vi "Test Dynamic Passing Method.vi"(8 "error in (no error)":errorcluster, 11 "Test Test Case in":refnum<class "Test Test Case.lvclass">) -> (0 "error out":errorcluster, 3 "Test Test Case out":refnum<class "Test Test Case.lvclass">)   [LabVIEW 2020, in "Test Test Case.lvclass"]
uses:
  Test Test Case.lvclass
  C:/Git/astemes-lunit/source/Framework/Test Case/LUnit Test Case.lvclass
  source/Framework/Test Case/LUnit Test Case.lvclass/LUnit Test Case.ctl
  source/Framework/Test Case/Private/SubVIs/Add test result.vi
  source/Framework/Test Case/Private/SubVIs/Set Assertion Type.vi
  source/Framework/Result Types/Case Result/Public/Record Assertion Result.vi
  source/Framework/Result Types/Method Result/Public/Aggregate Assertion Results.vi
  source/Framework/Result Types/Method Result/Private/Merge Status.vi
  source/Framework/Result Types/Method Result/Private/Concatenate result strings.vi
  source/Framework/Test Case/LUnit Test Case.lvclass
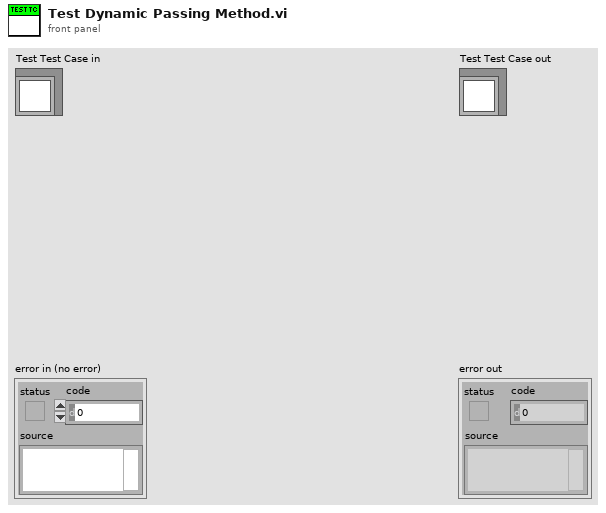
[diagram p1: front panel]
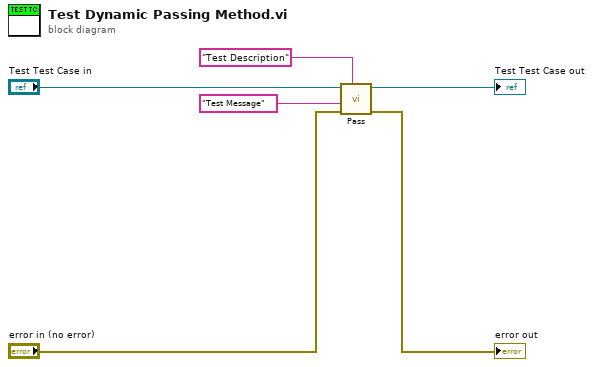
[diagram p0: block diagram]
diagram:
  n1 = call "Pass.vi"("Description"="Test Description", "error in (no error)"="error in (no error)", "Message"="Test Message", "LUnit Test Case In"="Test Test Case in") -> ("error out"=→"error out":errorcluster, "LUnit Test Case Out"=→"Test Test Case out":refnum<class "Test Test Case.lvclass">)  [unwired: 6 in]
